vi "Insyn.vi"(1 "txbuf":string) -> (0 "txbuf OUT":string)   [LabVIEW 2012]
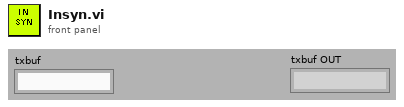
[diagram p1: front panel]
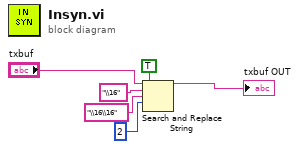
[diagram p0: block diagram]
diagram:
  n1 = Search and Replace String(replace all?=TRUE ("replace all? (F)"), input string="txbuf", search string="\\16", replace string="\\16\\16" ("replace string (\"\")"), offset=2 ("offset (0)")) -> (result string=→"txbuf OUT":string)  [unwired: 3 in, 3 out]
